vi "Select server.vi"(2 "Default Source":bool) -> (0 "DataSource":string)   [LabVIEW 2019]
uses:
  Process Controller 3.0/read-write.ctl
  Process Controller 3.0/ini interface.ctl
  DataServer/Server stats.ctl
panel:
  in  "new data source":bool
  out "Server Stats":T1[](array[typedef]) {"channel settings"."lower input limits" format="%.4f"; "channel settings"."upper input limits" format="%.4f"; "scan rate" format="%.2f"}
  in  "port":u16=6341
  in  "OK":bool
  in  "Data Sources":i32(listbox)
  # "Select the Data Source you would like to use."
  # "If the data source that you want to use is grayed out then the source is currently unavailable. \n\nDon't select a data source if you don't want to acquire data from a data server."
  # "Hz"
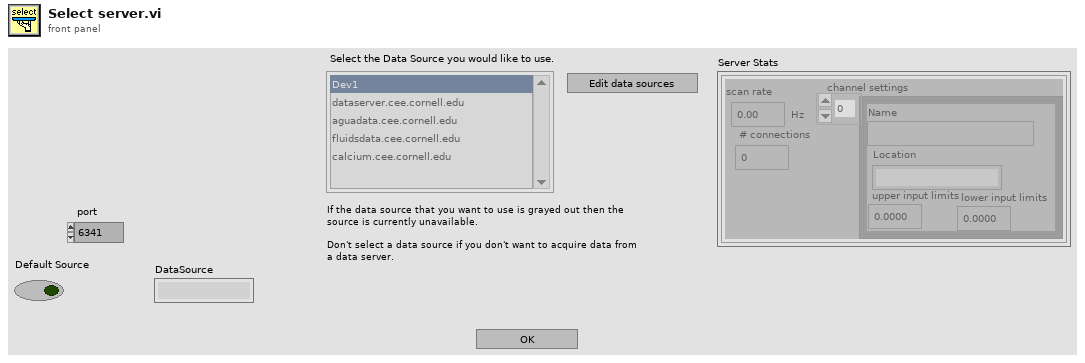
[diagram p1: front panel]
types:
  T1 = typedef "Server stats.ctl" = cluster{"scan rate":dbl, "# connections":i32, "channel settings":cluster{"Name":string, "upper input limits":sgl, "lower input limits":sgl, "Location":string}[]}
  T2 = typedef "ini interface.ctl" = enum16{"dataserver list", "dataserver", "com port", "stamp model", "Local Daq"}
  T3 = typedef "read-write.ctl" = enum16{"read", "write"}
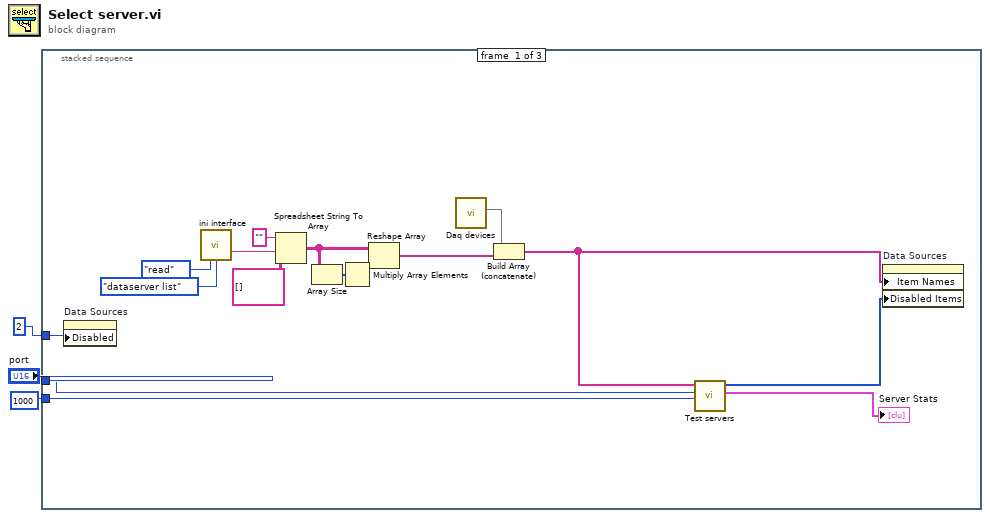
[diagram p0: block diagram]
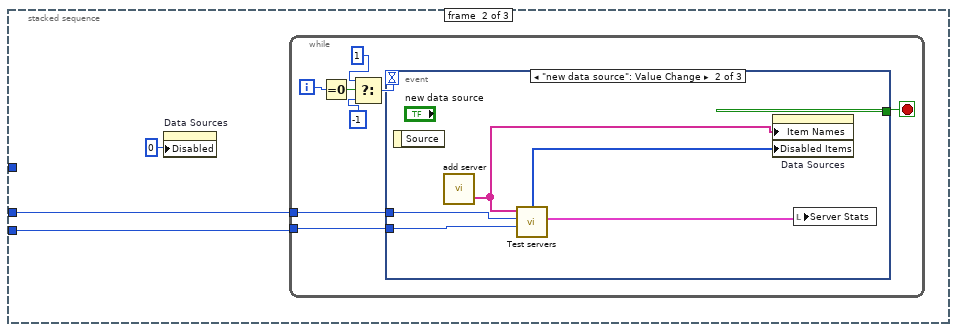
[diagram p2: hidden frame]
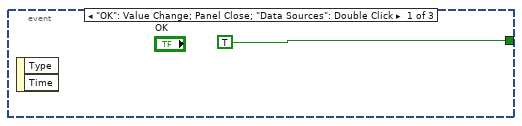
[diagram p3: hidden frame]
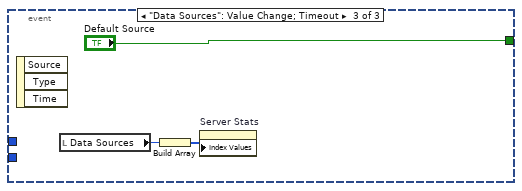
[diagram p4: hidden frame]
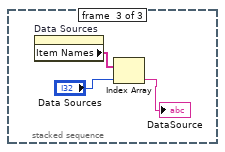
[diagram p5: hidden frame]
diagram:
  n1 = stacked-sequence {
    tunnel: "port" -> [w19 w22 _]
    tunnel: 1000 ("timeout ms (60000)") -> [w18 w21 _]
    tunnel: u8 2 ("Disabled") -> [w16 _ _]
    frame #0 {
      n2 = property on="Data Sources" class="LstBox (strict)"("Disabled"=w16) -> ()  [unwired: 2 in, 2 out]
      n3 = call "ini interface.vi"("direction"=read-write."read", "ini interface"=ini_interface."dataserver list") -> ("dataserver list out"=w13:string)  [unwired: 9 in, 4 out]
      n4 = Spreadsheet String To Array(format string="", spreadsheet string=w13, array type (2D Dbl)=string[][] []) -> (array=w9:string[][])  [unwired: 1 in]
      n5 = Array Size(array=w9) -> (size(s)=w8:i32[])
      n6 = Multiply Array Elements(1:w8) -> (0:w12:i32)
      n7 = Reshape Array(w9, w12) -> (w7:string[])
      n8 = call "Daq devices.vi"() -> (4:w6)  [unwired: 5 in, 5 out]
      n9 = Build Array (concatenate)(w6, w7) -> (w4:string[])
      n10 = call "Test servers.vi"("timeout ms (60000)"=w18, "port"=w19, "Server list"=w4) -> ("Server Stats"=→"Server Stats":T1[], "Disabled items"=w5:i32[])  [unwired: 7 in]
      n11 = property on="Data Sources" class="LstBox (strict)"("Item Names"=w4, "Disabled Items"=w5) -> ()  [unwired: 2 in, 2 out]
    }
    frame #1 {
      n12 = property on="Data Sources" class="LstBox (strict)"("Disabled"=u8 0) -> ()  [unwired: 2 in, 2 out]
      n13 = while {
        tunnel: w22 -> [w29]
        tunnel: w21 -> [w28]
        i -> [w27]
        stop <- w30 stop-if-true
        n14 = Equal To 0?(x=w27) -> (x = 0?=w26:bool)
        n15 = Select(t=1, s=w26, f=-1) -> (s? t:f=w23:i32)
        n16 = event shown="[1] \"new data source\": Value Change" {
          selector: _ -> [_ _ _]
          dyn-events: _ -> [_ _ _]
          timeout: w23 -> [_ _ _]
          tunnel: [TRUE ("OK") _ "Default Source"] -> w30
          tunnel: w29 -> [_ w36 _]
          tunnel: w28 -> [_ w35 _]
          event "OK": Value Change; Panel Close; "Data Sources": Double Click {
            n17 = event-data() -> ()  [unwired: 1 in, 2 out]
          }
          event "new data source": Value Change {
            n18 = event-data() -> ()  [unwired: 1 in, 1 out]
            n19 = call "add server.vi"() -> ("Server Array"=w32:string[])  [unwired: 2 in, 1 out]
            n20 = call "Test servers.vi"("timeout ms (60000)"=w35, "port"=w36, "Server list"=w32) -> ("Server Stats"=w34:T1[], "Disabled items"=w33:i32[])  [unwired: 7 in]
            n21 = property on="Data Sources" class="LstBox (strict)"("Item Names"=w32, "Disabled Items"=w33) -> ()  [unwired: 2 in, 2 out]
            n22 = local write "Server Stats"(w34) -> ()
          }
          event "Data Sources": Value Change; Timeout {
            n23 = event-data() -> ()  [unwired: 1 in, 3 out]
            n24 = local read "Data Sources"() -> (w39:i32)
            n25 = Build Array(w39) -> (w38:i32[])
            n26 = property on="Server Stats" class="Arr (strict)"("Index Values"=w38) -> ()  [unwired: 2 in, 2 out]
          }
        }
      }
    }
    frame #2 {
      n27 = property on="Data Sources" class="LstBox (strict)"() -> ("Item Names"=w42:string[])  [unwired: 2 in, 2 out]
      n28 = Index Array(array=w42, index="Data Sources") -> (element=→"DataSource":string)
    }
  }
